vi "XML-Read.vi"(8 "error in (no error)":errorcluster, 10 "Data":variant, 11 "XML File Path":path) -> (0 "error out":errorcluster, 2 "Data Out":variant, 3 "XML File Path(duplicate)":path)   [LabVIEW 2024]
uses:
  <vilib>/Utility/xml.llb/Read From XML File(string).vi
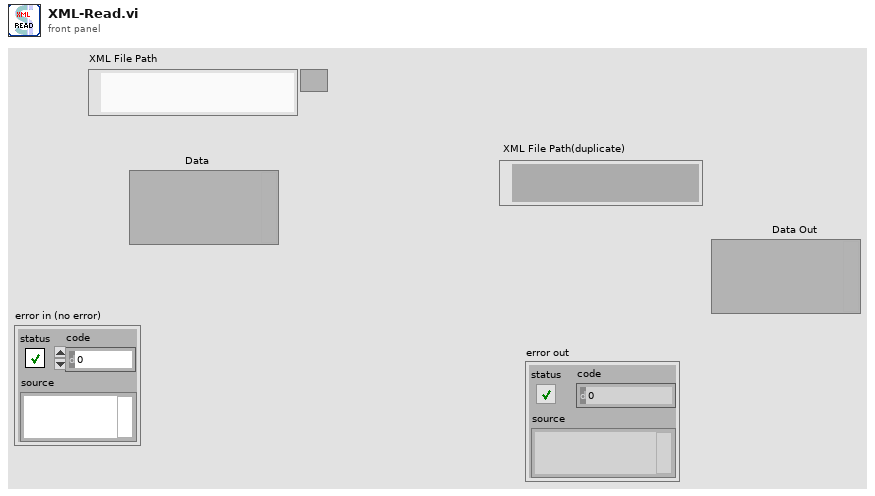
[diagram p1: front panel]
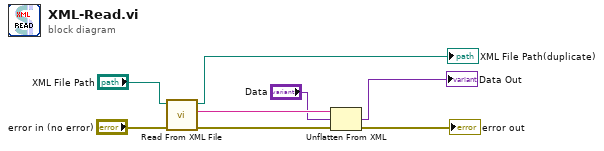
[diagram p0: block diagram]
diagram:
  n1 = call-poly <vilib>:"Read From XML File.vi"("error in (no error)"="error in (no error)", "XML File Path"="XML File Path") -> ("error out"=w7:errorcluster, "XML Elements"=w8:string, "XML File Path(duplicate)"=→"XML File Path(duplicate)":path)  [unwired: 7 in]
  n2 = Unflatten From XML(xml string=w8, type="Data", error in (no error)=w7) -> (value=→"Data Out":variant, error out=→"error out":errorcluster)
